vi "Is Deployed File Newer.vi"(8 "error in (no error)":errorcluster, 10 "Deployed Path":path, 11 "Template Path":path) -> (0 "error out":errorcluster, 2 "Deployed Newer?":bool)   [LabVIEW 2017]
doc: "Identifies if the deployed file is newer than the template file. Sets the boolean to true if it is"
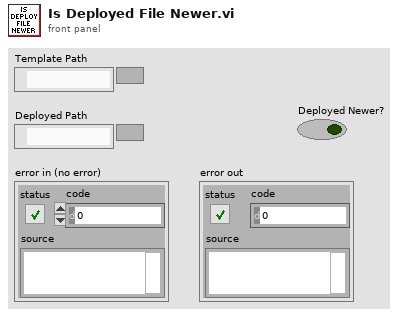
[diagram p1: front panel]
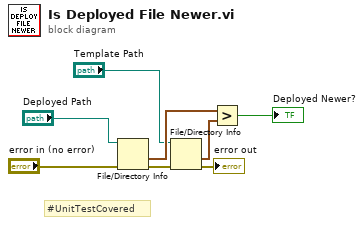
[diagram p0: block diagram]
diagram:
  # "#UnitTestCovered"
  n1 = File/Directory Info(path="Deployed Path", error in="error in (no error)") -> (last mod=w4:timestamp, error out=w7:errorcluster)  [unwired: 5 out]
  n2 = File/Directory Info(path="Template Path", error in=w7) -> (last mod=w3:timestamp, error out=→"error out":errorcluster)  [unwired: 5 out]
  n3 = Greater?(x=w4, y=w3) -> (0:→"Deployed Newer?":bool)
